vi "CycleAddGroup.vi"(11 "TreeControl输入":refnum<vi>) -> (1 "组名":string, 2 "添加的索引":i32, 3 "添加成功":bool)   [LabVIEW 2020, in "Curve Editor.lvlib"]
uses:
  Curve Editor.lvlib
panel:
  # "给树形列表添加组级标识，并输出组名"
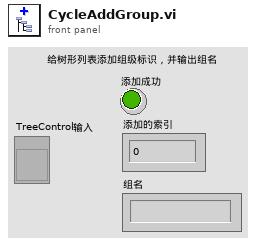
[diagram p1: front panel]
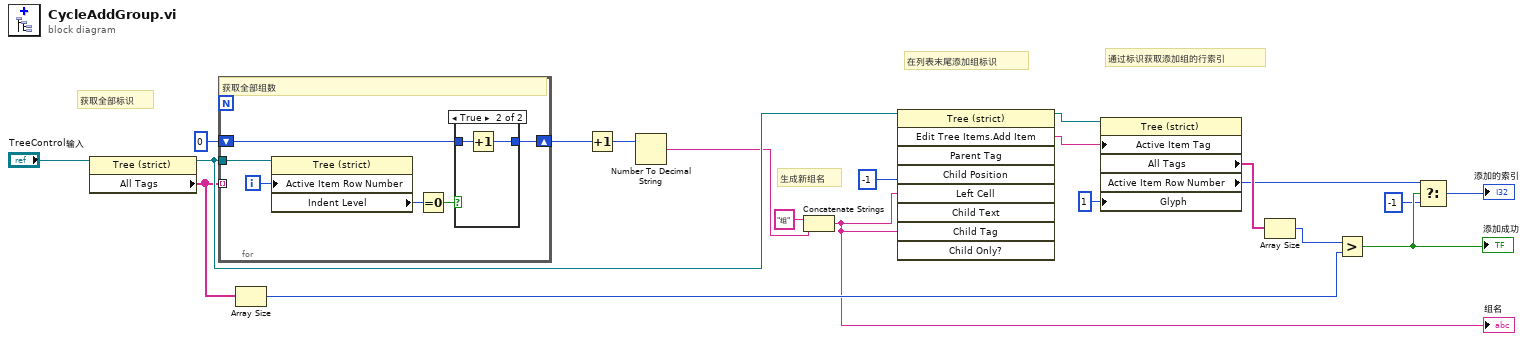
[diagram p0: block diagram]
diagram:
  # "通过标识获取添加组的行索引"
  # "在列表末尾添加组标识"
  # "生成新组名"
  # "获取全部标识"
  n1 = property class="Tree (strict)"(reference="TreeControl输入") -> (reference out=w19:refnum<vi>, "All Tags"=w12:string[])  [unwired: 1 in, 1 out]
  n2 = for {
    tunnel: w12 -> [_] mode=indexing
    tunnel: w19 -> [w26]
    shift-right: [w21] -> w17
    shift-left: 0 -> [w22]
    i -> [w25]
    # "获取全部组数"
    n3 = property class="Tree (strict)"(reference=w26, "Active Item Row Number"=w25) -> ("Indent Level"=w24:i32)  [unwired: 1 in, 2 out]
    n4 = Equal To 0?(x=w24) -> (x = 0?=w23:bool)
    n5 = case shown="True" w23 {
      tunnel: w22 -> [w27 w29]
      tunnel: [w27 w28] -> w21
      frame False {
      }
      frame True {
        n6 = Increment(x=w29) -> (x+1=w28:i32)
      }
    }
  }
  n7 = Array Size(array=w12) -> (size(s)=w8:i32)
  n8 = Increment(x=w17) -> (x+1=w20:i32)
  n9 = Number To Decimal String(number=w20) -> (decimal integer string=w18:string)  [unwired: 1 in]
  n10 = Concatenate Strings("组" ("字符串"), w18) -> (w3:string)
  "组名" <- w3
  n11 = invoke class="Tree (strict)" method="Edit Tree Items.Add Item"(reference=w19, "Child Position"=-1 ("子项位置"), "Left Cell"=w3, "Child Tag"=w3) -> (reference out=w2:refnum<vi>, "Edit Tree Items:Add Item"=w10:string)  [unwired: 5 in, 7 out]
  n12 = property class="Tree (strict)"(reference=w2, "Active Item Tag"=w10, "Glyph"=1 ("活动项:符号索引")) -> ("All Tags"=w11:string[], "Active Item Row Number"=w6:i32)  [unwired: 1 in, 2 out]
  n13 = Array Size(array=w11) -> (size(s)=w9:i32)
  n14 = Greater?(x=w9, y=w8) -> (0:w7:bool)
  "添加成功" <- w7
  n15 = Select(t=w6, s=w7, f=-1) -> (s? t:f=→"添加的索引":i32)
